vi "shutdown.vi"(8 "error in (no error)":errorcluster, 11 "ActiveMQBroker in":refnum<class "ActiveMQBroker.lvclass">) -> (0 "error out":errorcluster, 3 "ActiveMQBroker out":refnum<class "ActiveMQBroker.lvclass">)   [LabVIEW 2012, in "ActiveMQBroker.lvclass"]
uses:
  <userlib>/Common/Communication/ActiveMQ/ActiveMQBroker/ActiveMQBroker.lvclass
  <userlib>/Common/Communication/ActiveMQ/ActiveMQBroker/ActiveMQBroker.lvclass/ActiveMQBroker.ctl
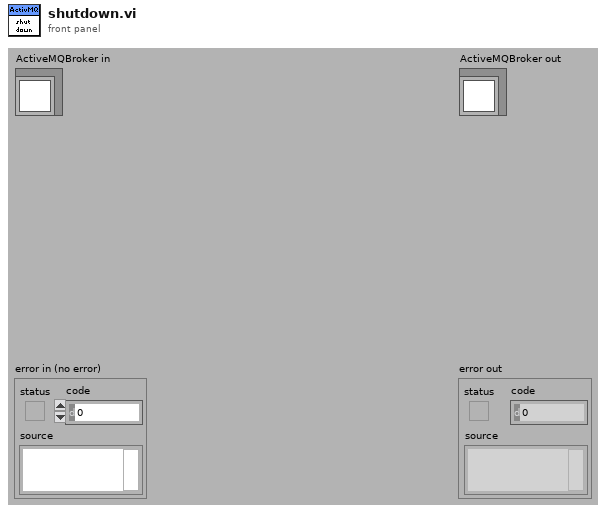
[diagram p1: front panel]
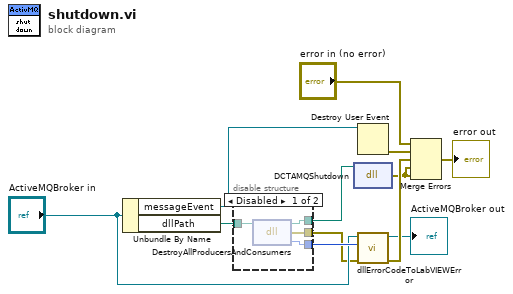
[diagram p0: block diagram]
diagram:
  n1 = Unbundle By Name("ActiveMQBroker in") -> ("messageEvent"=w9:refnum<user-event>, "dllPath"=w12:path)
  n2 = disable-structure shown="Disabled" {
    disable-tunnel: w12 -> [w16 w17]
    disable-tunnel: [w15 _] -> w11
    disable-tunnel: [w14 w17] -> w6
    disable-tunnel: [w13 _] -> w5
    frame Disabled {
      n3 = dll-call lib="C:/Documents and Settings/dan/My Documents/Lowell/source/DCT/trunk/Components/Common/ActiveMQ/DCTActiveMQHandler/C++ Source/DCTAMQ/Release/DCTAMQ.dll" fn="DestroyAllProducersAndConsumers"(path in=w16) -> (path out=w14:path, error out=w13:errorcluster, "return type"=w15:u32)  [unwired: 2 in]
    }
    frame Enabled {
    }
  }
  n4 = dll-call lib="?" fn="DCTAMQShutdown"(path in=w6) -> (error out=w1:errorcluster)  [unwired: 3 in, 1 out]
  n5 = Destroy User Event(user event=w9) -> (error out=w7:errorcluster)  [unwired: 1 in]
  n6 = call <userlib>:"dllErrorCodeToLabVIEWError.vi"("error in (no error)"=w5, "error code in"=w11, "ActiveMQBroker in"="ActiveMQBroker in") -> ("error out"=w4:errorcluster, "ActiveMQBroker out"=→"ActiveMQBroker out":refnum<class "ActiveMQBroker.lvclass">)  [unwired: 7 in]
  n7 = Merge Errors("error in (no error)", w7, w4, w1, w1) -> (→"error out":errorcluster)
